vi "GlobalVariable.vi"() -> ()   [LabVIEW 2020]
panel:
  out "connection ID":refnum<k5>
  out "连机状态":bool
  out "VI量程":bool[](array[boolean])
  out "V输出mbHR地址":u16[](array[numeric])
  out "电压输出":sgl[](array[numeric])
  in  "返回LOGO":bool
  in  "子VI退出":bool
  out "临界选数":dbl[][](array[numeric])
  in  "组件数":i32
  in  "有无接收":bool
  out "写完毕":bool
  out "读完毕":bool
  in  "电流":dbl[](array[numeric])
  in  "电压":dbl[](array[numeric])
  in  "计数率":u32[](array[numeric])
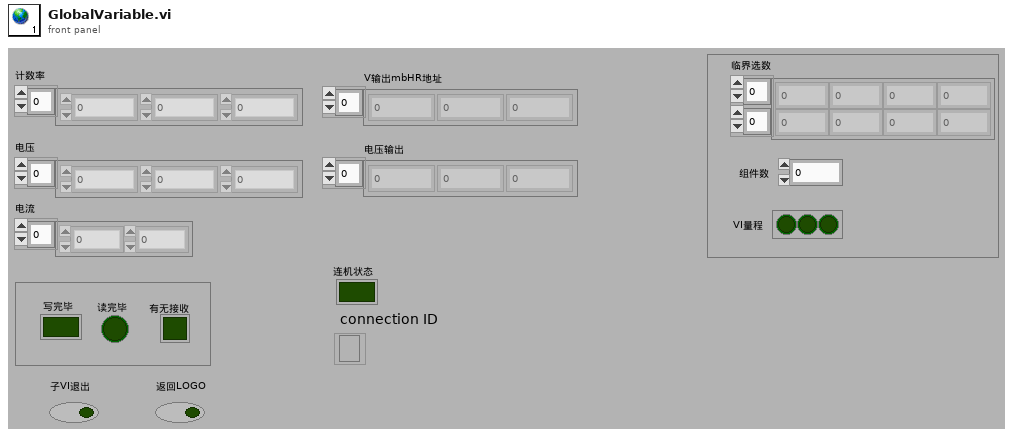
[diagram p1: front panel]
diagram:
